vi "ClsGetConnectionInfo.vi"(8 "error in (no error)":errorcluster, 11 "Connection In":u32) -> (0 "error out":errorcluster, 2 "Connection Info":string, 3 "Connection Out":u32)   [LabVIEW 2015]
doc: "Get Connection Info\n\nConnection In[Input]: the connection handle which is initially created by Open Connection subVI.\n\nConnection Info[Output]: string containing device connection information.\n\nConnection Out[Output]: the connection handle output which could be used for next subVI refering to the same connection."
uses:
  <vilib>/Utility/importsl/GetValueByPointer/datatype.ctl
  <vilib>/Utility/importsl/GetValueByPointer/GetValueByPointer.xnode
  dependent dlls/CHRocodileDLL.dll
  lvimptsl.dll
panel:
  out "Error Message":string
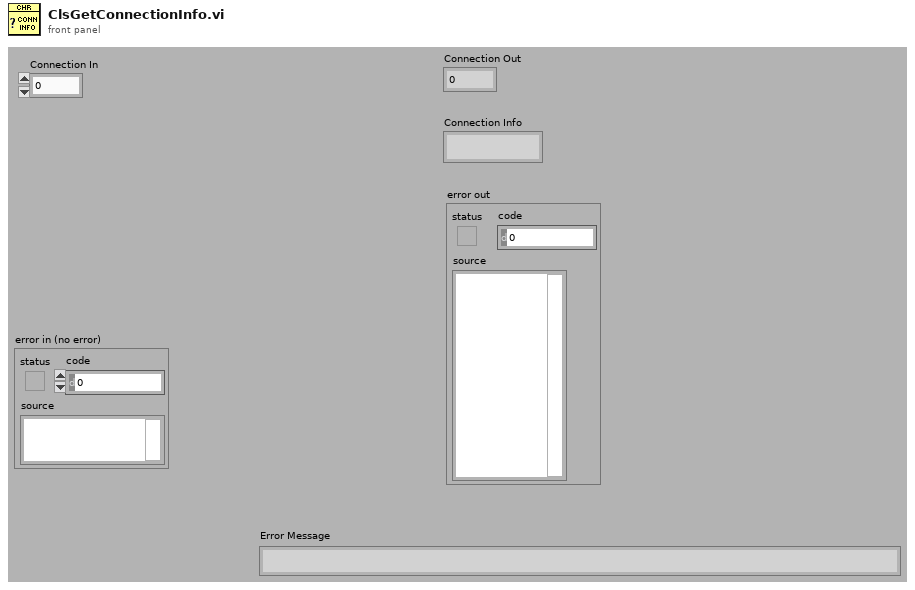
[diagram p1: front panel]
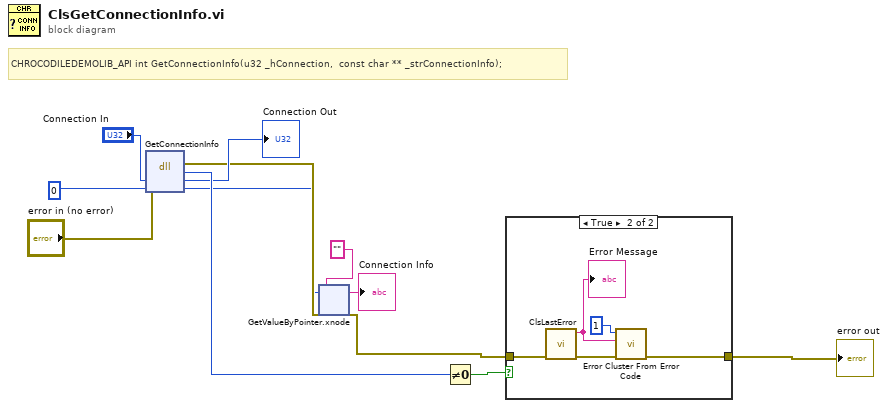
[diagram p0: block diagram]
diagram:
  # "CHROCODILEDEMOLIB_API int GetConnectionInfo(u32 _hConnection,  const char ** _strConnectionInfo);"
  n1 = dll-call lib="C:/Users/privat/Documents/ADP-SLA/Drop Impact Teststand/dependent dlls/CHRocodileDLL.*" fn="GetConnectionInfo"(error in="error in (no error)", "_hConnection"="Connection In", "_strConnectionInfo"=i64 0) -> (error out=w5:errorcluster, "return type"=w9:i32, "_hConnection"=→"Connection Out":u32, "_strConnectionInfo"=w3:i64)  [unwired: 2 in, 1 out]
  n2 = xnode "GetValueByPointer.xnode"("Pointer"=w3, "InputType"="" ("_pstrCmd 2"), "ErrorIn"=w5) -> ("Output"=→"Connection Info":string, "ErrorOut"=w4:errorcluster)  [unwired: 1 in]
  n3 = Not Equal To 0?(x=w9) -> (x != 0?=w11:bool)
  n4 = case shown="True" w11 {
    tunnel: [w13 w16] -> w10
    tunnel: w4 -> [w13 w15]
    frame False {
    }
    frame True {
      n5 = call "ClsLastError.vi"("error in (no error)"=w15) -> ("error out"=w14:errorcluster, "Error Message"=w18:string)  [unwired: 9 in]
      "Error Message" <- w18
      n6 = call <vilib>:"Error Cluster From Error Code.vi"("error in (no error)"=w14, "error message (\"\")"=w18, "error code (0)"=1) -> ("error out"=w16:errorcluster)  [unwired: 6 in]
    }
  }
  "error out" <- w10
